vi "Home.vi"() -> ()   [LabVIEW 2019]
uses:
  <vilib>/NI/Current Value Table/Type Defs/Single Tag.ctl
  <vilib>/NI/Current Value Table/Type Defs/Data Types.ctl
  <vilib>/Utility/miscctls.llb/LVDateTimeRec.ctl
  <vilib>/Utility/miscctls.llb/LVPointTypeDef.ctl
  <vilib>/NI/STM/TCP/Read Meta Data (TCP Ref).vi
  <vilib>/NI/STM/TCP/Get Connection Reference (TCP).vi
  <vilib>/NI/AMC/Create Single Message.vi
  <vilib>/NI/AMC/Update Message Routing Info.vi
  <vilib>/NI/AMC/Read Termination Message.vi
  <vilib>/NI/STM/TCP/Read Meta Data (TCP Clst).vi
  <vilib>/NI/AMC/Send Message.vi
  <vilib>/NI/AMC/Globals.vi
  <vilib>/NI/STM/TCP/Write Message (TCP).vi
  <vilib>/NI/STM/NI STM.lvlib
  <vilib>/NI/Current Value Table/Current Value Table.lvlib
  <vilib>/NI/AMC/AMC.lvlib
panel:
  out "Sulfuric Predip":dbl
  out "Current Step  6":i32 caption="Current Step"
  out "Current Step  5":i32 caption="Current Step"
  out "Current Step  4":i32 caption="Current Step"
  out "Current Step  3":i32 caption="Current Step"
  out "Current Step  2":i32 caption="Current Step"
  out "Current Step":i32
  out "Right Output On 6":bool caption="Right Output On"
  out "Left Output On 6":bool caption="Left Output On"
  out "Right Output On 5":bool caption="Right Output On"
  out "Left Output On 5":bool caption="Left Output On"
  out "Right Output On 4":bool caption="Right Output On"
  out "Left Output On 4":bool caption="Left Output On"
  out "Right Output On 3":bool caption="Right Output On"
  out "Left Output On 3":bool caption="Left Output On"
  out "Right Output On 2":bool caption="Right Output On"
  out "Left Output On 2":bool caption="Left Output On"
  out "Right Output On":bool
  out "Left Output On":bool
  out "Process 3 Accum A*hrs":dbl format="%.3f"
  out "Process 2 Accum A*hrs":dbl format="%.3f"
  out "Process 1 Accum A*hrs":dbl format="%.3f"
  in  "Reset All Chemical counters":bool
  out "Sulfuric P3":dbl
  out "Sulfuric P2":dbl
  out "Sulfuric P1":dbl
  out "Leveler P3":dbl
  out "Leveler P2":dbl
  out "Leveler P1":dbl
  out "Suppressor P3":dbl
  out "Suppressor P2":dbl
  out "Suppressor P1":dbl
  out "SPS P3":dbl
  out "SPS P2":dbl
  out "SPS P1":dbl
  out "Copper Oxide P3":dbl format="%.1f"
  out "Copper Oxide P2":dbl
  out "Copper Oxide P1":dbl format="%.1f"
  out "Since":timestamp
  in  "Reset DI Total counter":bool
  in  "LockOut HMI":bool
  out "User":string
  in  "Logout":bool
  in  "Login":bool
  out "Time Secs":dbl(knob) scale=0.0..12.0
  out "Time Mins":dbl(knob) scale=0.0..12.0
  out "Time Hours":dbl(knob) scale=0.0..12.0
  out "Liters DI Usage":dbl format="%#.1f"
  out "Main Electrical Cabinet T":dbl(slide) scale=10.0..55.0
  in  "Machine":bool
  in  "Run":bool
  in  "Basement 4":bool
  in  "Dryer":bool
  in  "Rinse 4":bool
  in  "Rinse 3":bool
  in  "Rinse 2":bool
  in  "Basement 3":bool
  in  "Basement 2":bool
  in  "Basement 1":bool
  in  "Plater 6":bool
  in  "Plater 5":bool
  in  "Plater 4":bool
  in  "Plater 3":bool
  in  "Plater 2":bool
  in  "Plater 1":bool
  in  "Predip":bool
  in  "Rinse 1":bool
  in  "Cleaner":bool
  in  "Etch":bool
  in  "Alarm History":i32(listbox)=-1
  out "# Alarms":u32
  in  "Alarms":i32(listbox)=-1
  in  "stop":bool
  in  "Reset Alarms":bool
  # "Module Selection"
  # "Do Not Operate"
  # "Warning"
  # "Plating Tank Status"
  # "Step"
  # "Left Anode"
  # "Right Anode"
  # "Tank 1"
  # "Tank 2"
  # "C"
  # "Tank 3"
  # "Tank 4"
  # "Tank 5"
  # "Tank 6"
  # "Copper"
  # "SPS"
  # "Suppressor"
  # "Leveler"
  # "Acid"
  # "Water Usage"
  # "Total Amp*Hrs"
  # "g"
  # "g"
  # "g"
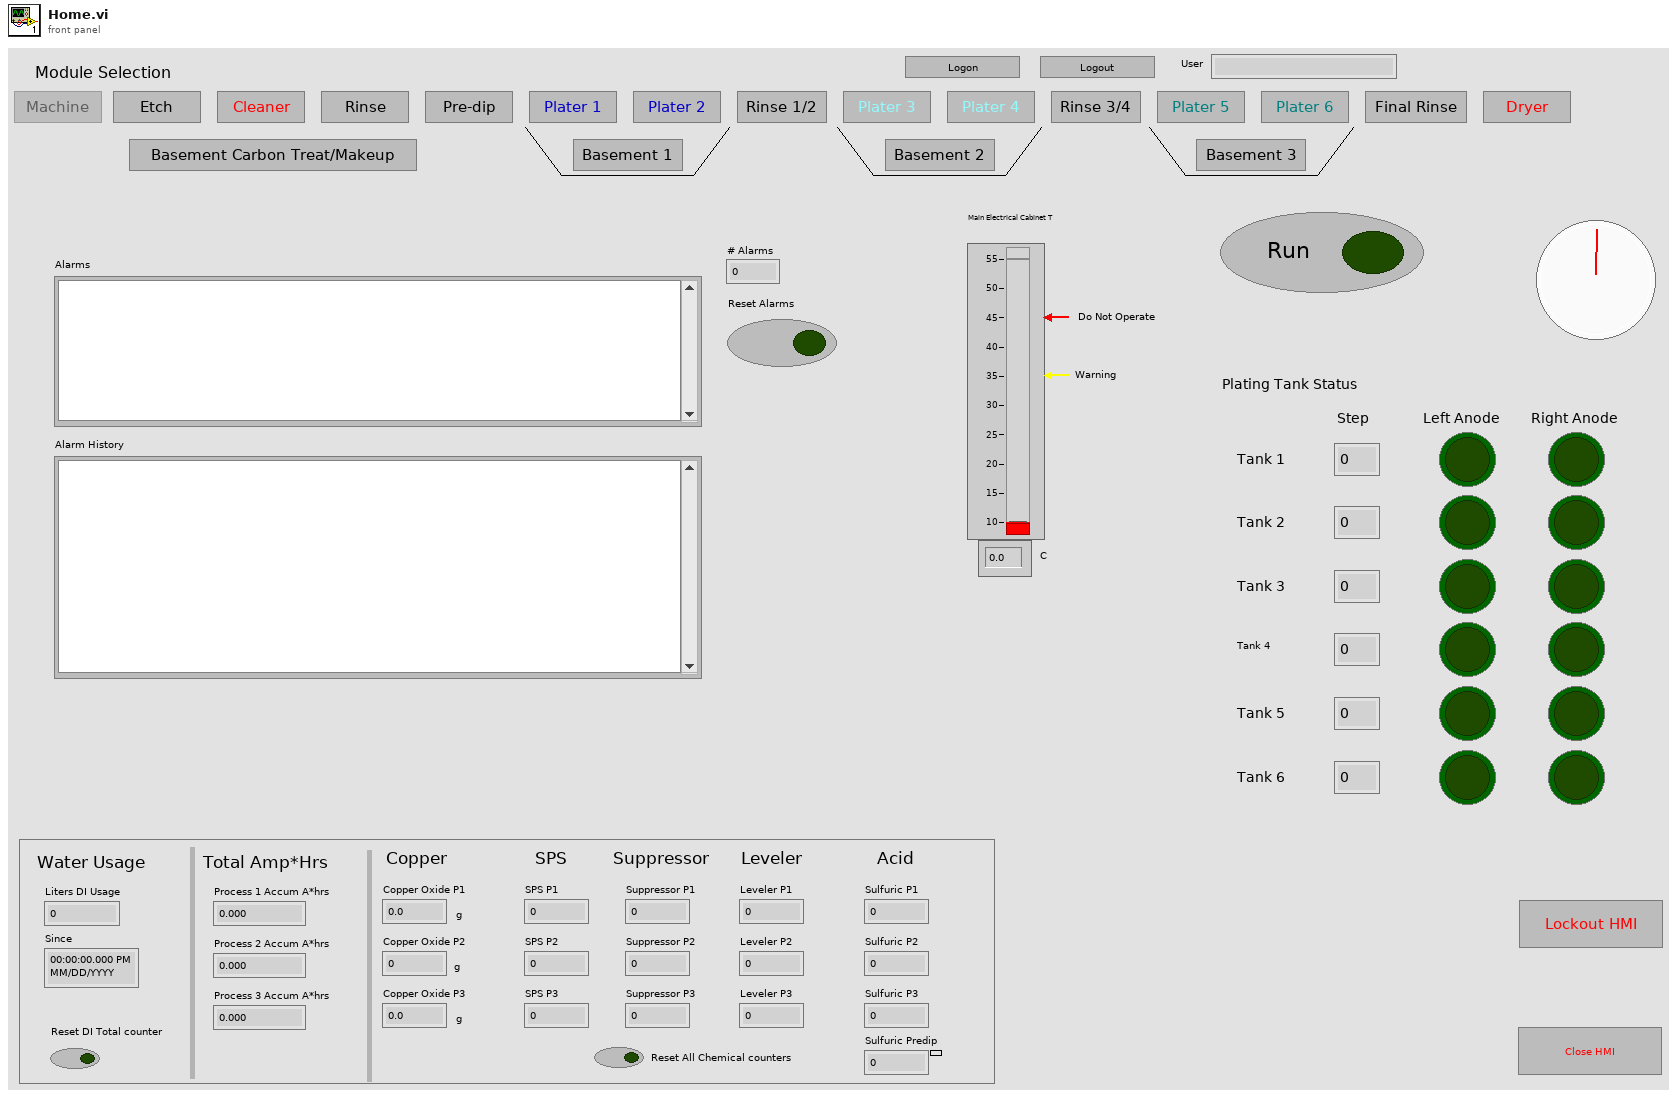
[diagram p1: front panel]
types:
  T1 = typedef "AMC.lvlib/Message Queue.ctl" = refnum<queue>
  T2 = typedef "NI STM.lvlib/TCP Connection Info.ctl" = cluster{"connection ID":refnum<k5>, "meta data":T3[]}
  T3 = typedef "NI STM.lvlib/MetaDataElement.ctl" = string
  T4 = cluster{"Shift":bool, "Ctrl":bool, "Alt":bool, "Cmd":bool, "Opt":bool}
  T5 = typedef "Current Value Table.lvlib/Single Tag.ctl" = cluster{"Data Type":T6, "Name":string, "Value":string, "Description":string}
  T6 = typedef "Current Value Table.lvlib/Data Types.ctl" = enum16{"Double", "Single", "I64", "I32", "I16", "I8", "U64", "U32", "U16", "U8", "String", "Boolean", "Array of U8", "Array of U16", "Array of U32", "Array of U64", "Array of I64", "Array of I32", "Array of I16", "Array of I8", "Array of Double", "Array of Single", "Array of Boolean", "Array of String"}
  T7 = enum8{"Enabled", "Disabled", "Disabled and Grayed Out"}
  T8 = typedef "LVPointTypeDef.ctl" = cluster{"Horizontal":i16, "Vertical":i16}
  T9 = typedef "LVDateTimeRec.ctl" = cluster{"fractional second":dbl, "second":i32, "minute":i32, "hour":i32, "day of month":i32, "month":i32, "year":i32, "day of week":i32, "day of year":i32, "DST":i32}
  T10 = cluster{"second":i32, "minute":i32, "hour":i32, "day of month":i32, "month":i32, "year":i32, "day of week":i32, "day of year":i32, "is DST":i32}
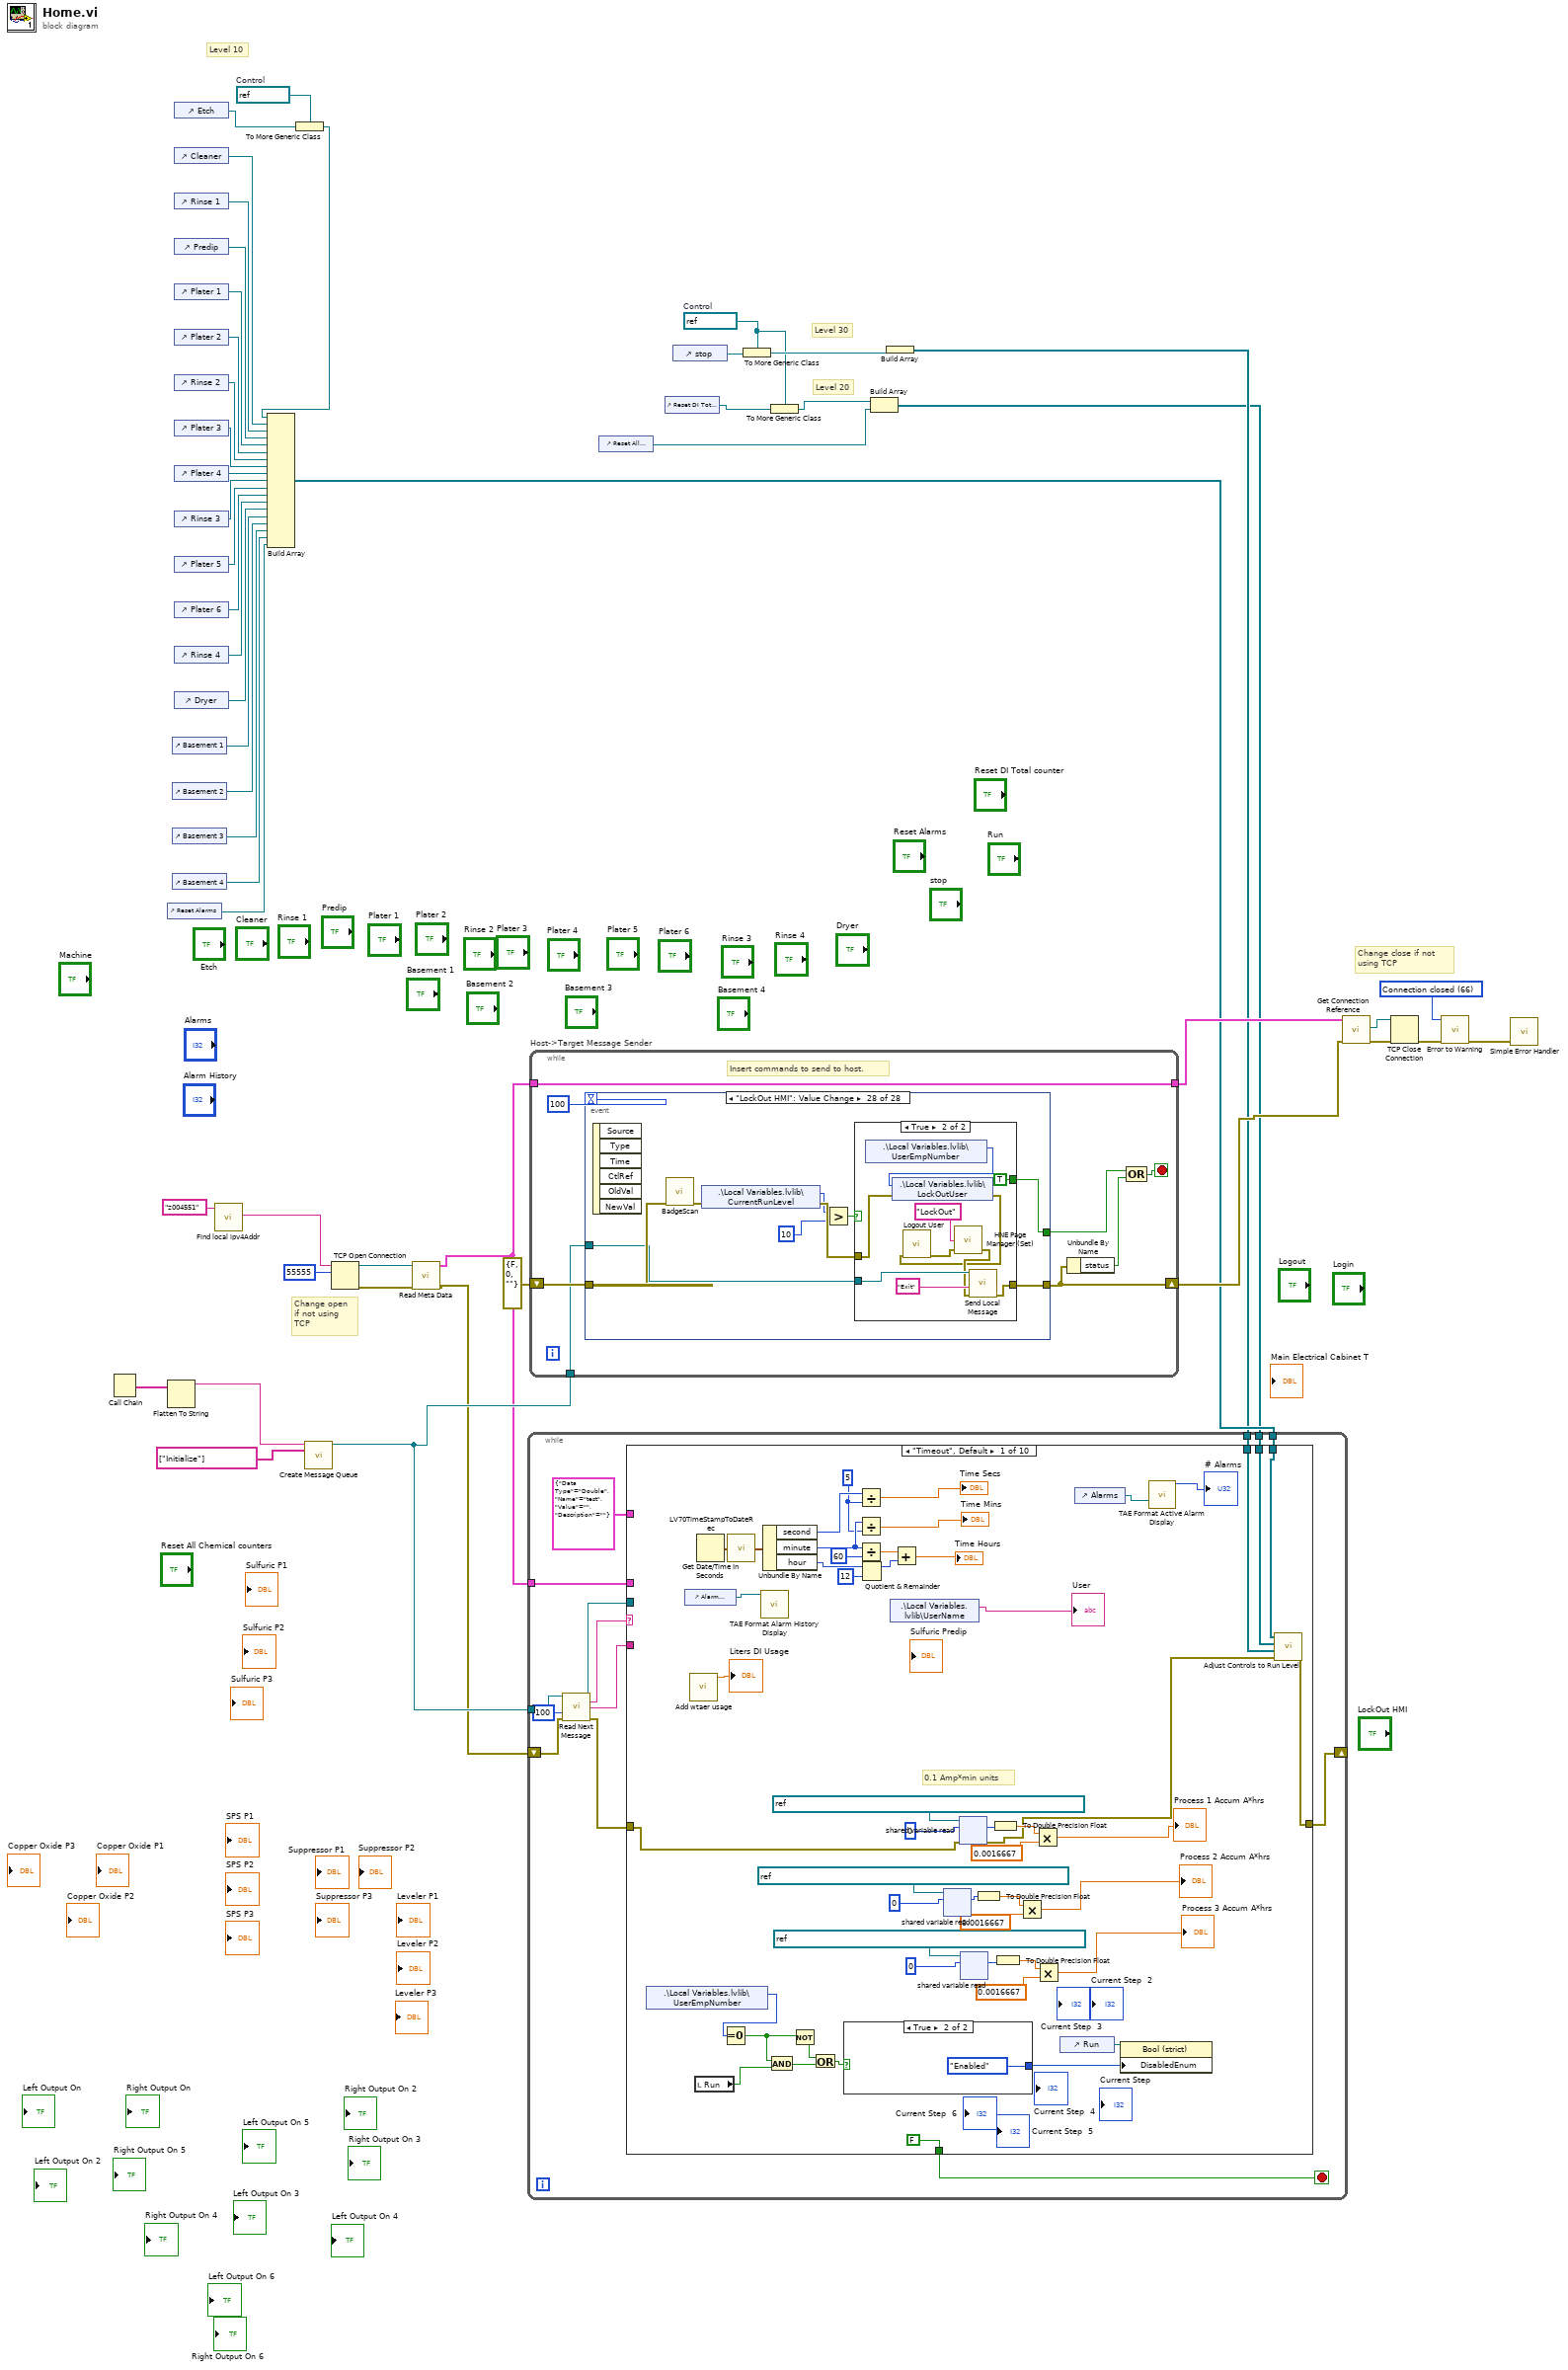
[diagram p0: block diagram]
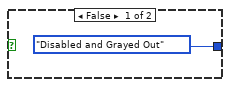
[diagram p2: hidden frame]
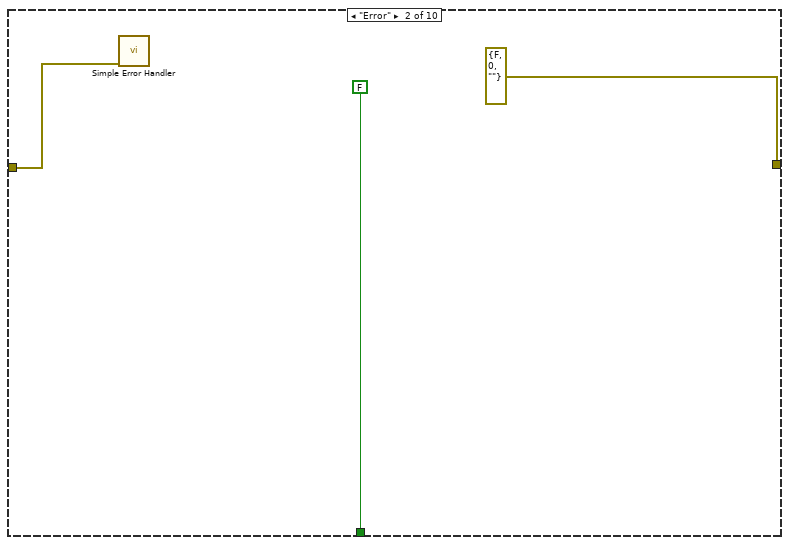
[diagram p3: hidden frame]
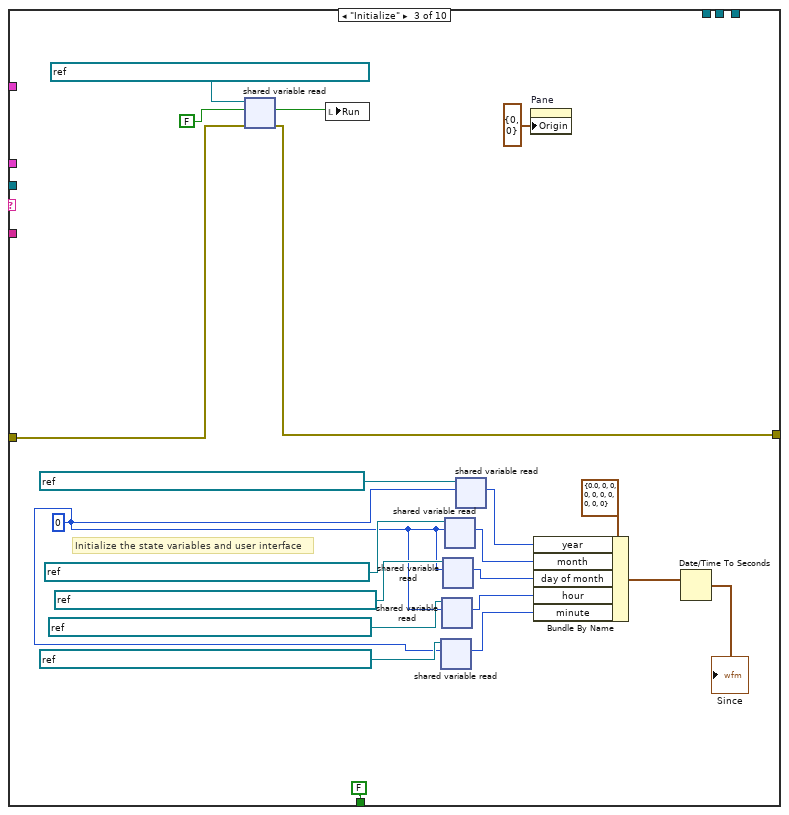
[diagram p4: hidden frame]
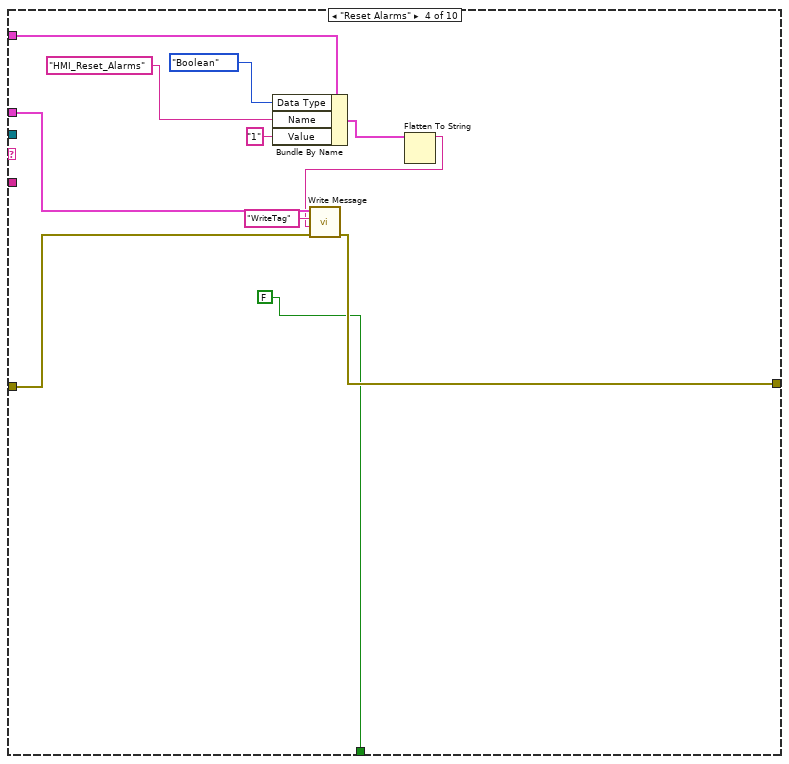
[diagram p5: hidden frame]
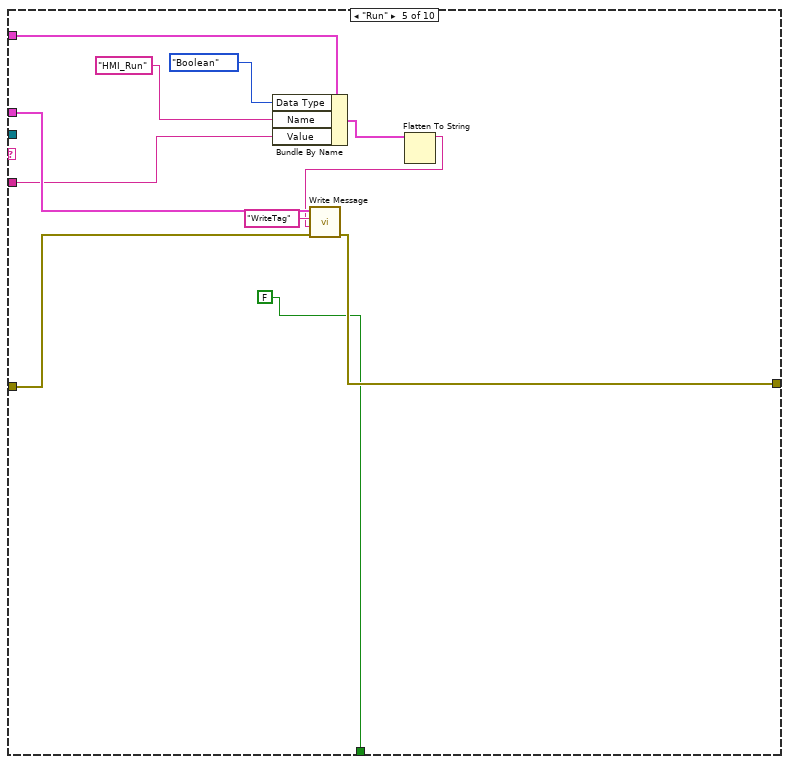
[diagram p6: hidden frame]
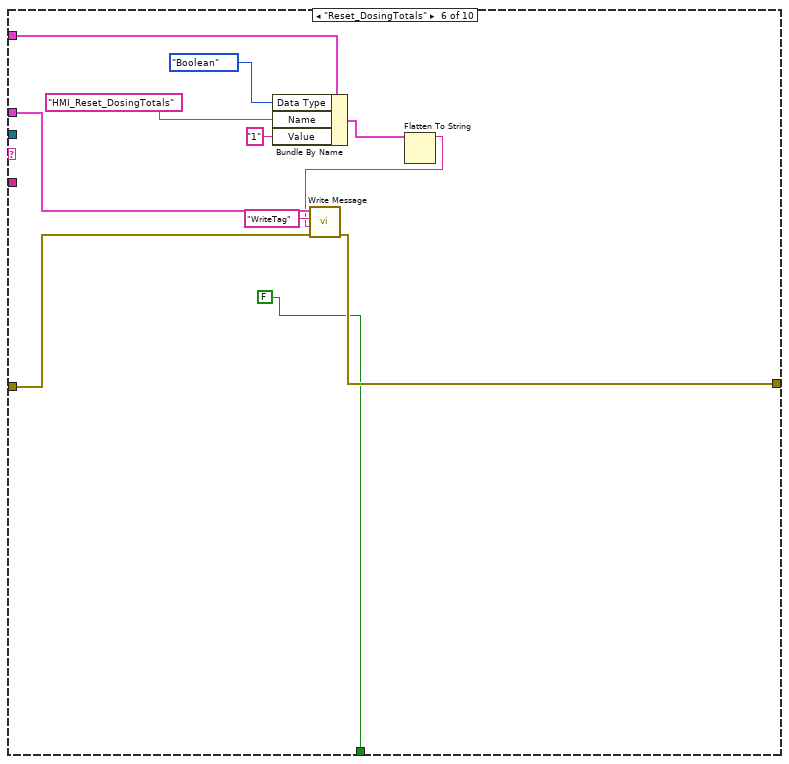
[diagram p7: hidden frame]
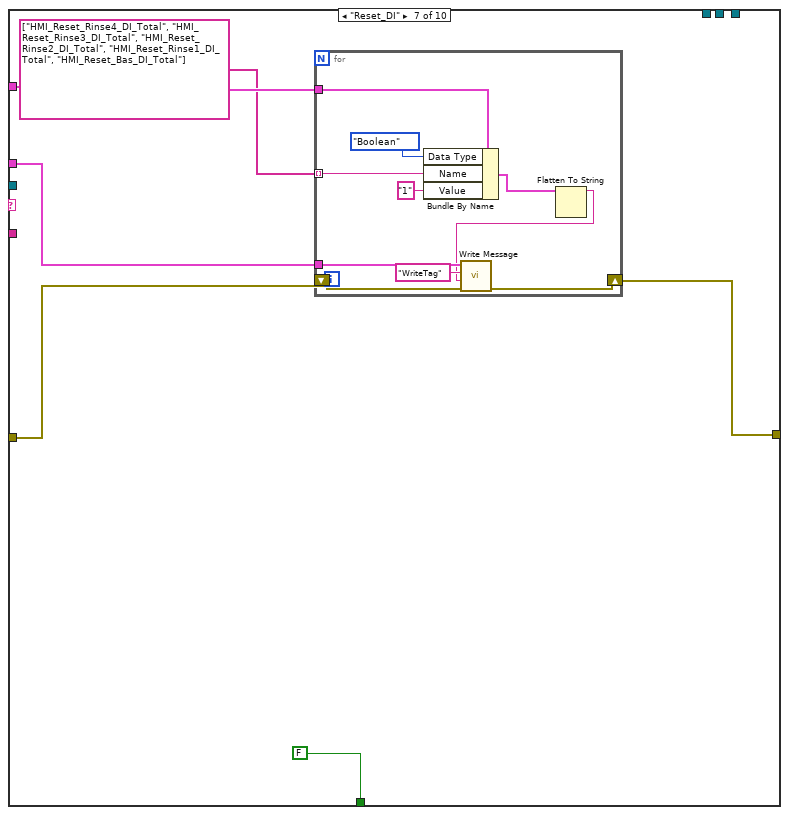
[diagram p8: hidden frame]
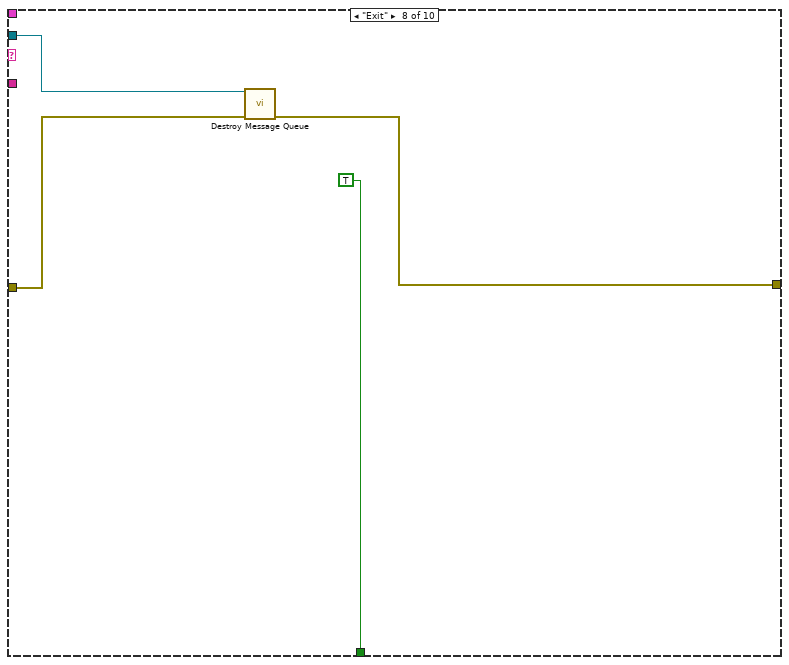
[diagram p9: hidden frame]
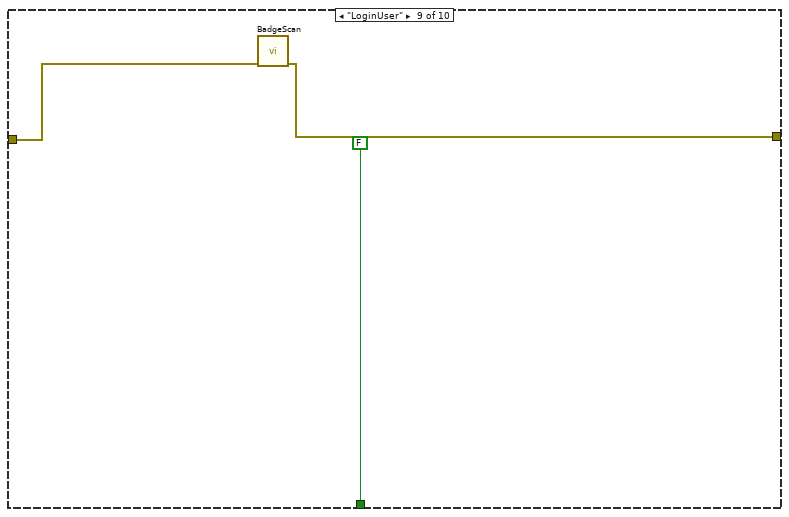
[diagram p10: hidden frame]
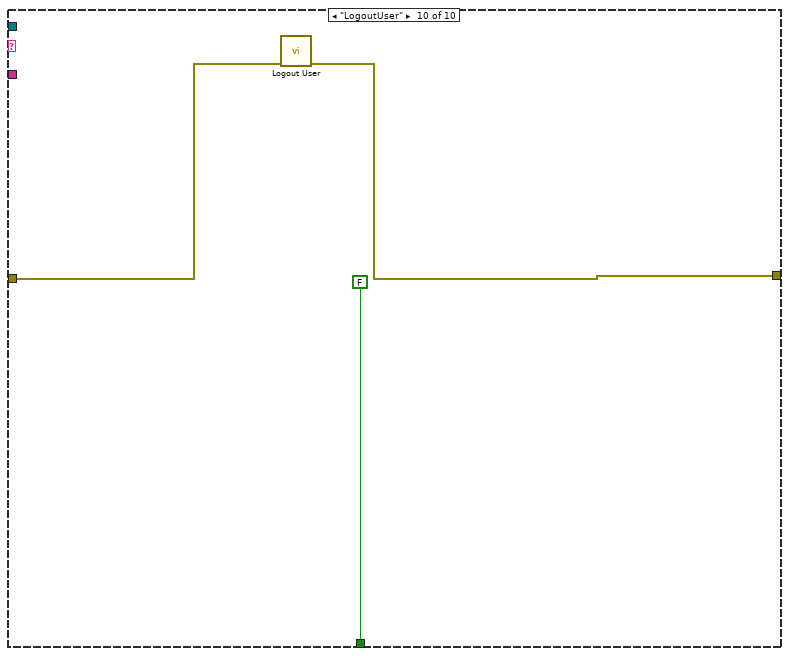
[diagram p11: hidden frame]
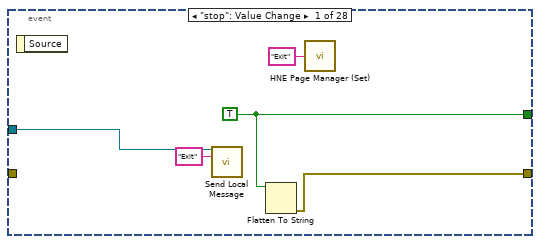
[diagram p12: hidden frame]
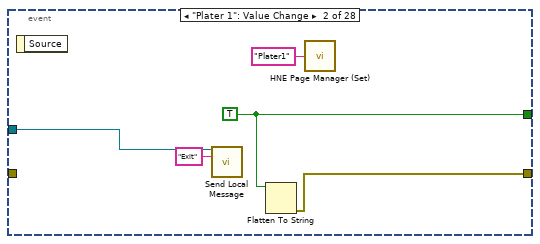
[diagram p13: hidden frame]
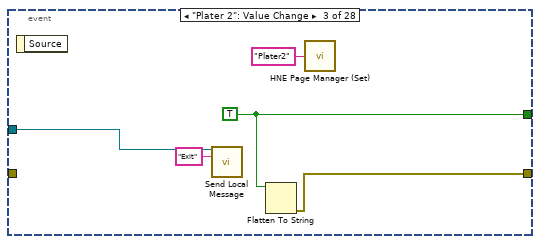
[diagram p14: hidden frame]
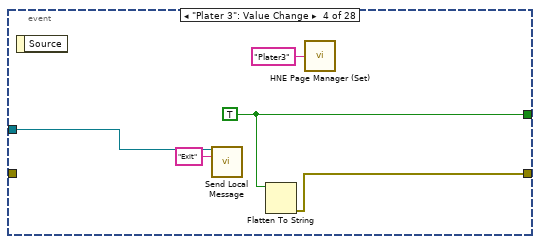
[diagram p15: hidden frame]
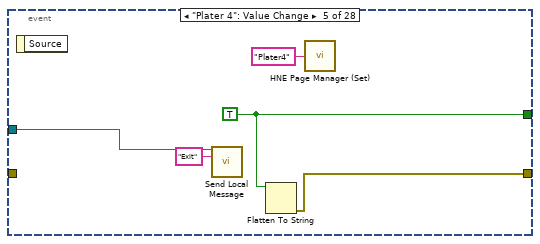
[diagram p16: hidden frame]
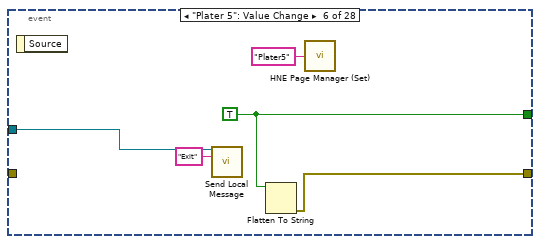
[diagram p17: hidden frame]
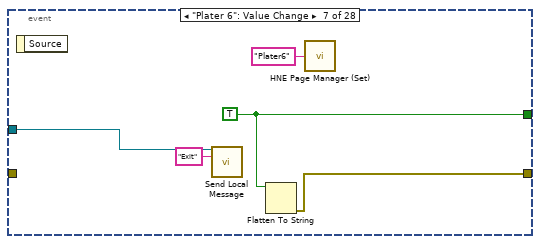
[diagram p18: hidden frame]
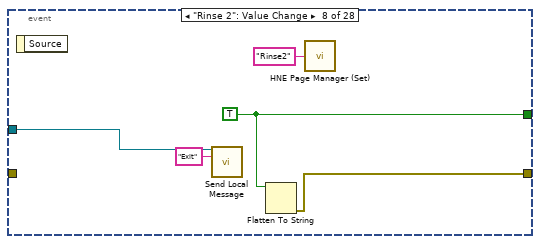
[diagram p19: hidden frame]
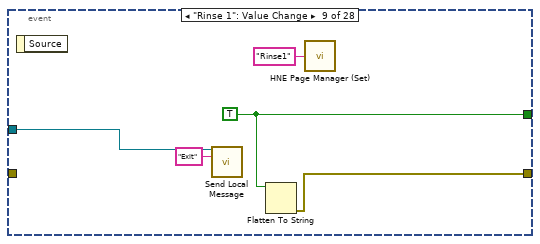
[diagram p20: hidden frame]
diagram:
  w8 = refnum<vi> refnum  # Control
  w4 = refnum<vi> refnum  # Control
  w48 = 66 items=["No Error", "Argument Error", "Memory Full", "Out of Zone", "End of File", "File Already Open", "Generic File IO Error", "File Not Found", "File Permission Error", "Disk Full", "Duplicate Path", "Too Many Files Open", "Not Enabled", "Resource File Not Found", "Cannot Add Resource", "Resource Not Found", "Image Not Found", "Image Memory Error", "Pen Does Not Exist", "Config Bad Type", "Config Token Not Found", "Config Parse Error", "Config Memory Error", "Bad External Code Format", "Bad External Code Offset", "External Code Not Present", "Null Window", "Destroy Window Mixup", "Null Menu", "Print Aborted", "Bad Print Record", "Print Driver Error", "Windows Error During Print", "Memory Error During Print", "Print Dialog Error", "Generic Print Error", "Invalid Device Refnum", "Device Not Found", "Device Parameter Error", "Device Unit Error", "Can't Open Device", "Device Call Aborted", "Generic Error", "Cancelled By User", "Object ID Too Low", "Object ID Too High", "Object Not In Heap", "Unknown Heap", "Bad DefProc ID", "DefProc Not In Table", "Message Out Of Range", "Null Method", "Unknown Message", "Manager Call Not Supported", "Bad address", "Connection In progress", "Connection timed out", "Connection is already in progress", "Network attribute not supported", "Network error", "Address in use", "System out of memory", "Connection aborted", "Connection refused", "Connection is not connected", "Connection is already connected", "Connection closed", "Initialize error (interapplication manager)", "Bad occurrence", "Wait on unbound occurrence handler", "Occurrence queue overflow", "Bad path", "Semaphore not signaled", "Unrecognized type (interapplication manager)"] ("1st Error to Convert")
  # "Level 10"
  # "Level 20"
  # "Level 30"
  # "Change close if not using TCP"
  # "Change open if not using TCP"
  n1 = Call Chain() -> (call chain=w40:string[])
  n2 = control-ref of="Reset Alarms"() -> (w12:refnum<vi>)
  n3 = Flatten To String(anything=w40) -> (data string=w39:string)  [unwired: 3 in, 2 out]
  n4 = control-ref of="Basement 1"() -> (w17:refnum<vi>)
  n5 = control-ref of="Basement 2"() -> (w16:refnum<vi>)
  n6 = control-ref of="Basement 3"() -> (w15:refnum<vi>)
  n7 = control-ref of="Basement 4"() -> (w14:refnum<vi>)
  n8 = control-ref of="Etch"() -> (w7:refnum<vi>)
  n9 = control-ref of="Cleaner"() -> (w30:refnum<vi>)
  n10 = control-ref of="Rinse 1"() -> (w29:refnum<vi>)
  n11 = control-ref of="Predip"() -> (w28:refnum<vi>)
  n12 = control-ref of="Plater 1"() -> (w27:refnum<vi>)
  n13 = control-ref of="Plater 2"() -> (w26:refnum<vi>)
  n14 = control-ref of="Rinse 2"() -> (w25:refnum<vi>)
  n15 = control-ref of="Plater 3"() -> (w24:refnum<vi>)
  n16 = control-ref of="Plater 4"() -> (w23:refnum<vi>)
  n17 = control-ref of="Rinse 3"() -> (w22:refnum<vi>)
  n18 = control-ref of="Plater 5"() -> (w21:refnum<vi>)
  n19 = control-ref of="Plater 6"() -> (w20:refnum<vi>)
  n20 = control-ref of="Rinse 4"() -> (w19:refnum<vi>)
  n21 = control-ref of="Dryer"() -> (w18:refnum<vi>)
  n22 = call "Find local ipv4Addr.vi"("MachineToFind"="z004551") -> ("name"=w34:string)  [unwired: 9 in, 1 out]
  n23 = To More Generic Class(target class=w8, reference=w7) -> (generic class reference=w6:refnum<vi>)
  n24 = Build Array(w6, w30, w29, w28, w27, w26, w25, w24, w23, w22, w21, w20, w19, w18, w17, w16, w15, w14, w12) -> (w13:refnum<vi>[])
  n25 = call <vilib>:"Create Message Queue.vi"("message queue name"=w39, "initial message names"=string[] ["Initialize"] ("initial message values")) -> ("message queue out"=w37:T1)  [unwired: 12 in, 1 out]
  n26 = TCP Open Connection(address=w34, remote port or service name=u16 55555 ("remote port")) -> (connection ID=w44:refnum<k5>, error out=w43:errorcluster)  [unwired: 1 in, 2 out]
  n27 = call-poly <vilib>:"Read Meta Data.vi"("error in"=w43, "connection ID"=w44) -> ("error out"=w36:errorcluster, "connection info out"=w32:T2)  [unwired: 7 in, 1 out]
  n28 = while "Host->Target Message Sender" {
    shift-right: [w54] -> w42
    shift-left: errorcluster {"status"=FALSE, "code"=0, "source"=""} ("error out") -> [w57]
    tunnel: [w50] -> w41
    tunnel: w37 -> [w51]
    tunnel: w32 -> [w50]
    stop <- w55 stop-if-true
    # "Insert commands to send to host."
    n29 = event shown="[27] \"LockOut HMI\": Value Change" {
      selector: _ -> [_ _ _ _ _ _ _ _ _ _ _ _ _ _ _ _ _ _ _ _ _ _ _ _ _ _ _ _]
      dyn-events: _ -> [_ _ _ _ _ _ _ _ _ _ _ _ _ _ _ _ _ _ _ _ _ _ _ _ _ _ _ _]
      timeout: 100 -> [_ _ _ _ _ _ _ _ _ _ _ _ _ _ _ _ _ _ _ _ _ _ _ _ _ _ _ _]
      tunnel: w57 -> [_ _ _ _ _ _ _ _ _ _ _ _ _ _ _ _ _ _ _ w154 w161 w166 w175 w183 w187 w190 w191 w205]
      tunnel: [w62 w67 w72 w77 w82 w87 w92 w97 w102 w107 w112 w117 w122 w127 w132 w137 w142 w147 w152 _ _ _ _ _ _ _ _ w197] -> w53
      tunnel: [w61 w66 w71 w76 w81 w86 w91 w96 w101 w106 w111 w116 w121 w126 w131 w136 w141 w146 w151 w153 w160 w165 w174 w182 w186 w190 w191 w200] -> w54
      tunnel: w51 -> [w59 w64 w69 w74 w79 w84 w89 w94 w99 w104 w109 w114 w119 w124 w129 w134 w139 w144 w149 w156 w163 w167 w176 w185 w189 _ _ w201]
      event "stop": Value Change {
        w62 = TRUE ("stop")
        n30 = event-data() -> ()  [unwired: 2 out]
        n31 = call <vilib>:"Send Local Message.vi"("message queue in"=w59, "message name"="Exit") -> ()  [unwired: 11 in, 3 out]
        n32 = Flatten To String(anything=w62) -> (error out=w61:errorcluster)  [unwired: 2 in, 3 out]
        n33 = call <userlib>:"HNE Page Manager (Set).vi"("Next Page"="Exit") -> ()  [unwired: 4 in, 1 out]
      }
      event "Plater 1": Value Change {
        w67 = TRUE ("stop")
        n34 = event-data() -> ()  [unwired: 2 out]
        n35 = call <vilib>:"Send Local Message.vi"("message queue in"=w64, "message name"="Exit") -> ()  [unwired: 11 in, 3 out]
        n36 = Flatten To String(anything=w67) -> (error out=w66:errorcluster)  [unwired: 2 in, 3 out]
        n37 = call <userlib>:"HNE Page Manager (Set).vi"("Next Page"="Plater1") -> ()  [unwired: 4 in, 1 out]
      }
      event "Plater 2": Value Change {
        w72 = TRUE ("stop")
        n38 = event-data() -> ()  [unwired: 2 out]
        n39 = call <vilib>:"Send Local Message.vi"("message queue in"=w69, "message name"="Exit") -> ()  [unwired: 11 in, 3 out]
        n40 = Flatten To String(anything=w72) -> (error out=w71:errorcluster)  [unwired: 2 in, 3 out]
        n41 = call <userlib>:"HNE Page Manager (Set).vi"("Next Page"="Plater2") -> ()  [unwired: 4 in, 1 out]
      }
      event "Plater 3": Value Change {
        w77 = TRUE ("stop")
        n42 = event-data() -> ()  [unwired: 2 out]
        n43 = call <vilib>:"Send Local Message.vi"("message queue in"=w74, "message name"="Exit") -> ()  [unwired: 11 in, 3 out]
        n44 = Flatten To String(anything=w77) -> (error out=w76:errorcluster)  [unwired: 2 in, 3 out]
        n45 = call <userlib>:"HNE Page Manager (Set).vi"("Next Page"="Plater3") -> ()  [unwired: 4 in, 1 out]
      }
      event "Plater 4": Value Change {
        w82 = TRUE ("stop")
        n46 = event-data() -> ()  [unwired: 2 out]
        n47 = call <vilib>:"Send Local Message.vi"("message queue in"=w79, "message name"="Exit") -> ()  [unwired: 11 in, 3 out]
        n48 = Flatten To String(anything=w82) -> (error out=w81:errorcluster)  [unwired: 2 in, 3 out]
        n49 = call <userlib>:"HNE Page Manager (Set).vi"("Next Page"="Plater4") -> ()  [unwired: 4 in, 1 out]
      }
      event "Plater 5": Value Change {
        w87 = TRUE ("stop")
        n50 = event-data() -> ()  [unwired: 2 out]
        n51 = call <vilib>:"Send Local Message.vi"("message queue in"=w84, "message name"="Exit") -> ()  [unwired: 11 in, 3 out]
        n52 = Flatten To String(anything=w87) -> (error out=w86:errorcluster)  [unwired: 2 in, 3 out]
        n53 = call <userlib>:"HNE Page Manager (Set).vi"("Next Page"="Plater5") -> ()  [unwired: 4 in, 1 out]
      }
      event "Plater 6": Value Change {
        w92 = TRUE ("stop")
        n54 = event-data() -> ()  [unwired: 2 out]
        n55 = call <vilib>:"Send Local Message.vi"("message queue in"=w89, "message name"="Exit") -> ()  [unwired: 11 in, 3 out]
        n56 = Flatten To String(anything=w92) -> (error out=w91:errorcluster)  [unwired: 2 in, 3 out]
        n57 = call <userlib>:"HNE Page Manager (Set).vi"("Next Page"="Plater6") -> ()  [unwired: 4 in, 1 out]
      }
      event "Rinse 2": Value Change {
        w97 = TRUE ("stop")
        n58 = event-data() -> ()  [unwired: 2 out]
        n59 = call <vilib>:"Send Local Message.vi"("message queue in"=w94, "message name"="Exit") -> ()  [unwired: 11 in, 3 out]
        n60 = Flatten To String(anything=w97) -> (error out=w96:errorcluster)  [unwired: 2 in, 3 out]
        n61 = call <userlib>:"HNE Page Manager (Set).vi"("Next Page"="Rinse2") -> ()  [unwired: 4 in, 1 out]
      }
      event "Rinse 1": Value Change {
        w102 = TRUE ("stop")
        n62 = event-data() -> ()  [unwired: 2 out]
        n63 = call <vilib>:"Send Local Message.vi"("message queue in"=w99, "message name"="Exit") -> ()  [unwired: 11 in, 3 out]
        n64 = Flatten To String(anything=w102) -> (error out=w101:errorcluster)  [unwired: 2 in, 3 out]
        n65 = call <userlib>:"HNE Page Manager (Set).vi"("Next Page"="Rinse1") -> ()  [unwired: 4 in, 1 out]
      }
      event "Rinse 3": Value Change {
        w107 = TRUE ("stop")
        n66 = event-data() -> ()  [unwired: 2 out]
        n67 = call <vilib>:"Send Local Message.vi"("message queue in"=w104, "message name"="Exit") -> ()  [unwired: 11 in, 3 out]
        n68 = Flatten To String(anything=w107) -> (error out=w106:errorcluster)  [unwired: 2 in, 3 out]
        n69 = call <userlib>:"HNE Page Manager (Set).vi"("Next Page"="Rinse3") -> ()  [unwired: 4 in, 1 out]
      }
      event "Rinse 4": Value Change {
        w112 = TRUE ("stop")
        n70 = event-data() -> ()  [unwired: 2 out]
        n71 = call <vilib>:"Send Local Message.vi"("message queue in"=w109, "message name"="Exit") -> ()  [unwired: 11 in, 3 out]
        n72 = Flatten To String(anything=w112) -> (error out=w111:errorcluster)  [unwired: 2 in, 3 out]
        n73 = call <userlib>:"HNE Page Manager (Set).vi"("Next Page"="Rinse4") -> ()  [unwired: 4 in, 1 out]
      }
      event "Dryer": Value Change {
        w117 = TRUE ("stop")
        n74 = event-data() -> ()  [unwired: 2 out]
        n75 = call <vilib>:"Send Local Message.vi"("message queue in"=w114, "message name"="Exit") -> ()  [unwired: 11 in, 3 out]
        n76 = Flatten To String(anything=w117) -> (error out=w116:errorcluster)  [unwired: 2 in, 3 out]
        n77 = call <userlib>:"HNE Page Manager (Set).vi"("Next Page"="Dryer") -> ()  [unwired: 4 in, 1 out]
      }
      event "Predip": Value Change {
        w122 = TRUE ("stop")
        n78 = event-data() -> ()  [unwired: 2 out]
        n79 = call <vilib>:"Send Local Message.vi"("message queue in"=w119, "message name"="Exit") -> ()  [unwired: 11 in, 3 out]
        n80 = Flatten To String(anything=w122) -> (error out=w121:errorcluster)  [unwired: 2 in, 3 out]
        n81 = call <userlib>:"HNE Page Manager (Set).vi"("Next Page"="Predip") -> ()  [unwired: 4 in, 1 out]
      }
      event "Cleaner": Value Change {
        w127 = TRUE ("stop")
        n82 = event-data() -> ()  [unwired: 2 out]
        n83 = call <vilib>:"Send Local Message.vi"("message queue in"=w124, "message name"="Exit") -> ()  [unwired: 11 in, 3 out]
        n84 = Flatten To String(anything=w127) -> (error out=w126:errorcluster)  [unwired: 2 in, 3 out]
        n85 = call <userlib>:"HNE Page Manager (Set).vi"("Next Page"="Clean") -> ()  [unwired: 4 in, 1 out]
      }
      event "Etch": Value Change {
        w132 = TRUE ("stop")
        n86 = event-data() -> ()  [unwired: 2 out]
        n87 = call <vilib>:"Send Local Message.vi"("message queue in"=w129, "message name"="Exit") -> ()  [unwired: 11 in, 3 out]
        n88 = Flatten To String(anything=w132) -> (error out=w131:errorcluster)  [unwired: 2 in, 3 out]
        n89 = call <userlib>:"HNE Page Manager (Set).vi"("Next Page"="Etch") -> ()  [unwired: 4 in, 1 out]
      }
      event "Basement 1": Value Change {
        w137 = TRUE ("stop")
        n90 = event-data() -> ()  [unwired: 2 out]
        n91 = call <vilib>:"Send Local Message.vi"("message queue in"=w134, "message name"="Exit") -> ()  [unwired: 11 in, 3 out]
        n92 = Flatten To String(anything=w137) -> (error out=w136:errorcluster)  [unwired: 2 in, 3 out]
        n93 = call <userlib>:"HNE Page Manager (Set).vi"("Next Page"="Basement1") -> ()  [unwired: 4 in, 1 out]
      }
      event "Basement 2": Value Change {
        w142 = TRUE ("stop")
        n94 = event-data() -> ()  [unwired: 2 out]
        n95 = call <vilib>:"Send Local Message.vi"("message queue in"=w139, "message name"="Exit") -> ()  [unwired: 11 in, 3 out]
        n96 = Flatten To String(anything=w142) -> (error out=w141:errorcluster)  [unwired: 2 in, 3 out]
        n97 = call <userlib>:"HNE Page Manager (Set).vi"("Next Page"="Basement2") -> ()  [unwired: 4 in, 1 out]
      }
      event "Basement 3": Value Change {
        w147 = TRUE ("stop")
        n98 = event-data() -> ()  [unwired: 2 out]
        n99 = call <vilib>:"Send Local Message.vi"("message queue in"=w144, "message name"="Exit") -> ()  [unwired: 11 in, 3 out]
        n100 = Flatten To String(anything=w147) -> (error out=w146:errorcluster)  [unwired: 2 in, 3 out]
        n101 = call <userlib>:"HNE Page Manager (Set).vi"("Next Page"="Basement3") -> ()  [unwired: 4 in, 1 out]
      }
      event "Basement 4": Value Change {
        w152 = TRUE ("stop")
        n102 = event-data() -> ()  [unwired: 2 out]
        n103 = call <vilib>:"Send Local Message.vi"("message queue in"=w149, "message name"="Exit") -> ()  [unwired: 11 in, 3 out]
        n104 = Flatten To String(anything=w152) -> (error out=w151:errorcluster)  [unwired: 2 in, 3 out]
        n105 = call <userlib>:"HNE Page Manager (Set).vi"("Next Page"="Basement4") -> ()  [unwired: 4 in, 1 out]
      }
      event "Reset Alarms": Value Change {
        n106 = event-data() -> ()  [unwired: 2 out]
        n107 = call <vilib>:"Send Local Message.vi"("message queue in"=w156, "message name"="Reset Alarms", "error in"=w154) -> ("error out"=w153:errorcluster)  [unwired: 10 in, 2 out]
      }
      event "Run": Value Change {
        n108 = event-data() -> ("NewVal"=w159:bool)  [unwired: 1 out]
        n109 = Boolean To (0,1)(Boolean=w159) -> (0, 1=w158:i16)
        n110 = Number To Decimal String(number=w158) -> (decimal integer string=w157:string)  [unwired: 1 in]
        n111 = call <vilib>:"Send Local Message.vi"("message queue in"=w163, "message name"="Run", "message value"=w157, "error in"=w161) -> ("error out"=w160:errorcluster)  [unwired: 9 in, 2 out]
      }
      event "Reset DI Total counter": Value Change {
        n112 = event-data() -> ("NewVal"=w164:bool)  [unwired: 1 out]
        n113 = case shown="True" w164 {
          tunnel: w167 -> [_ w172]
          tunnel: w166 -> [w168 w170]
          tunnel: [w168 w169] -> w165
          frame False {
          }
          frame True {
            n114 = call <vilib>:"Send Local Message.vi"("message queue in"=w172, "message name"="Reset_DI", "error in"=w170) -> ("error out"=w169:errorcluster)  [unwired: 10 in, 2 out]
          }
        }
      }
      event "Reset All Chemical counters": Value Change {
        n115 = event-data() -> ("NewVal"=w173:bool)  [unwired: 1 out]
        n116 = case shown="True" w173 {
          tunnel: w176 -> [_ w181]
          tunnel: w175 -> [w177 w179]
          tunnel: [w177 w178] -> w174
          frame False {
          }
          frame True {
            n117 = call <vilib>:"Send Local Message.vi"("message queue in"=w181, "message name"="Reset_DosingTotals", "error in"=w179) -> ("error out"=w178:errorcluster)  [unwired: 10 in, 2 out]
          }
        }
      }
      event "Login": Value Change {
        n118 = event-data() -> ()  [unwired: 7 out]
        n119 = call <vilib>:"Send Local Message.vi"("message queue in"=w185, "message name"="LoginUser", "error in"=w183) -> ("error out"=w182:errorcluster)  [unwired: 10 in, 2 out]
      }
      event "Logout": Value Change {
        n120 = event-data() -> ()  [unwired: 7 out]
        n121 = call <vilib>:"Send Local Message.vi"("message queue in"=w189, "message name"="LogoutUser", "error in"=w187) -> ("error out"=w186:errorcluster)  [unwired: 10 in, 2 out]
      }
      event Timeout {
        n122 = event-data() -> ()  [unwired: 2 out]
      }
      event Mouse Down? {
        n123 = event-data() -> ("Button"=w196:u16, "Mods"=w195:cluster{"Double Click":bool, "Menu Key":bool}, "PlatMods"=w194:T4)  [unwired: 6 out]
        n124 = Get Date/Time In Seconds() -> (seconds since 1Jan1904=w192:timestamp)
        n125 = shared-variable ".\\Local Variables.lvlib\\LastLogonTime"(w192) -> ()  [unwired: 1 in, 1 out]
        n126 = event-data("Button"=w196, "Mods"=w195, "PlatMods"=w194, "Discard?"=FALSE) -> ()  [unwired: 1 in, 1 out]
      }
      event "LockOut HMI": Value Change {
        n127 = event-data() -> ()  [unwired: 7 out]
        n128 = call "BadgeScan.vi"("error in"=w205) -> ("error out"=w204:errorcluster)  [unwired: 10 in]
        n129 = shared-variable ".\\Local Variables.lvlib\\CurrentRunLevel"(error in=w204) -> (w199:i32, error out=w202:errorcluster)
        n130 = Greater?(x=w199, y=10 ("x")) -> (0:w203:bool)
        n131 = case shown="True" w203 {
          tunnel: w202 -> [w207 w210]
          tunnel: w201 -> [_ w216]
          tunnel: [w207 w214] -> w200
          tunnel: [FALSE ("stop") TRUE ("stop")] -> w197
          frame False {
          }
          frame True {
            n132 = shared-variable ".\\Local Variables.lvlib\\UserEmpNumber"() -> (w211:i32)  [unwired: 1 in, 1 out]
            n133 = shared-variable ".\\Local Variables.lvlib\\LockOutUser"(w211, error in=w210) -> (error out=w209:errorcluster)
            n134 = call "Logout User.vi"("error in (no error)"=w209) -> ("error out"=w212:errorcluster)  [unwired: 10 in]
            n135 = call <userlib>:"HNE Page Manager (Set).vi"("error in (no error)"=w212, "Next Page"="LockOut") -> ("error out"=w213:errorcluster)  [unwired: 3 in]
            n136 = call <vilib>:"Send Local Message.vi"("message queue in"=w216, "message name"="Exit", "error in"=w213) -> ("error out"=w214:errorcluster)  [unwired: 10 in, 2 out]
          }
        }
      }
    }
    n137 = Unbundle By Name(w54) -> ("status"=w52:bool)
    n138 = Compound Arithmetic op=OR(w53, w52) -> (w55:bool)
  }
  n139 = control-ref of="Reset All Chemical counters"() -> (w1:refnum<vi>)
  n140 = control-ref of="Reset DI Total counter"() -> (w5:refnum<vi>)
  n141 = control-ref of="stop"() -> (w11:refnum<vi>)
  n142 = To More Generic Class(target class=w4, reference=w11) -> (generic class reference=w10:refnum<vi>)
  n143 = To More Generic Class(target class=w4, reference=w5) -> (generic class reference=w3:refnum<vi>)
  n144 = Build Array(w3, w1) -> (w2:refnum<vi>[])
  n145 = Build Array(w10) -> (w9:refnum<vi>[])
  n146 = while {
    tunnel: w37 -> [w231]
    tunnel: w32 -> [w228]
    shift-right: [w226] -> _
    shift-left: w36 -> [w222]
    tunnel: w13 -> [w220]
    tunnel: w9 -> [w219]
    tunnel: w2 -> [w218]
    stop <- w225 stop-if-true
    n147 = call <vilib>:"Read Next Message.vi"("message queue in"=w231, "timeout (1 ms)"=100, "error in"=w222) -> ("message queue out"=w224:T1, "message name"=w229:string, "message value"=w227:string, "error out"=w221:errorcluster)  [unwired: 5 in, 4 out]
    n148 = case shown="\"Timeout\", Default" w229 {
      tunnel: w228 -> [_ _ _ w318 w329 w340 w347 _ _ _]
      tunnel: w227 -> [_ _ _ _ w320 _ _ _ _ _]
      tunnel: w221 -> [w233 w285 w305 w317 w328 w339 w346 w359 w364 w366]
      tunnel: [w234 errorcluster {"status"=FALSE, "code"=0, "source"=""} ("error out") w304 w316 w327 w338 w345 w358 w363 w365] -> w226
      tunnel: [FALSE FALSE FALSE FALSE FALSE FALSE FALSE TRUE FALSE FALSE] -> w225
      tunnel: w224 -> [_ _ _ _ _ _ _ w360 _ _]
      tunnel: T5 {"Data Type"=enum."Double", "Name"="test", "Value"="", "Description"=""} ("Tag") -> [_ _ _ w310 w322 w333 w344 _ _ _]
      tunnel: w220 -> [w255 _ _ _ _ _ _ _ _ _]
      tunnel: w219 -> [w254 _ _ _ _ _ _ _ _ _]
      tunnel: w218 -> [w253 _ _ _ _ _ _ _ _ _]
      frame "Timeout", Default {
        w269 = 5 ("y")
        # "0.1 Amp*min units"
        n149 = shared-variable ".\\Local Variables.lvlib\\UserEmpNumber"() -> (w263:i32)  [unwired: 1 in, 1 out]
        n150 = control-ref of="Alarm History"() -> (w279:refnum<vi>)
        n151 = call "Add wtaer usage.vi"() -> ("Numeric"=→"Liters DI Usage":dbl)  [unwired: 11 in]
        n152 = local read "Run"() -> (w262:bool)
        n153 = Get Date/Time In Seconds() -> (seconds since 1Jan1904=w268:timestamp)
        n154 = Equal To 0?(x=w263) -> (x = 0?=w261:bool)
        n155 = call <vilib>:"LV70TimeStampToDateRec.vi"("time stamp"=w268) -> ("date time rec"=w277:T10)
        n156 = call <userlib>:"TAE Format Alarm History Display.vi"("List Box Ref"=w279) -> ()  [unwired: 13 in, 2 out]
        n157 = Unbundle By Name(w277) -> ("second"=w276:i32, "minute"=w275:i32, "hour"=w272:i32)
        n158 = And(x=w261, y=w262) -> (x .and. y?=w258:bool)
        n159 = Not(x=w261) -> (.not. x?=w259:bool)
        n160 = Or(x=w259, y=w258) -> (x .or. y?=w260:bool)
        n161 = case shown="True" w260 {
          tunnel: [T7."Disabled and Grayed Out" ("Disabled") T7."Enabled" ("Disabled")] -> w256
          frame False {
          }
          frame True {
          }
        }
        n162 = Divide(x=w276, y=w269) -> (x/y=→"Time Secs":dbl)
        n163 = Divide(x=w275, y=w269) -> (x/y=→"Time Mins":dbl)
        n164 = Divide(x=w275, y=60) -> (x/y=w273:dbl)
        n165 = Quotient & Remainder(x=w272, y=12) -> (x-y*floor(x/y)=w270:i32)  [unwired: 1 out]
        n166 = shared-variable ".\\Local Variables.lvlib\\UserName"() -> (→"User":string)  [unwired: 1 in, 1 out]
        n167 = Add(x=w273, y=w270) -> (x+y=→"Time Hours":dbl)
        n168 = shared-variable-read(refnum<k21> "ni.var.psp://z004551/CDL0100 ReadTags/Proc2_TotalAmpMin" ("shared variable refnum in"), 0) -> (w238:i32)  [unwired: 1 in, 3 out]
        n169 = shared-variable-read(refnum<k21> "ni.var.psp://z004551/CDL0100 ReadTags/Proc1_TotalAmpMin" ("shared variable refnum in"), w233, 0) -> (w232:errorcluster, w240:i32)  [unwired: 2 out]
        n170 = shared-variable-read(refnum<k21> "ni.var.psp://z004551/CDL0100 ReadTags/Proc3_TotalAmpMin" ("shared variable refnum in"), 0) -> (w237:i32)  [unwired: 1 in, 3 out]
        n171 = To Double Precision Float(number=w238) -> (double precision float=w235:dbl)
        n172 = To Double Precision Float(number=w240) -> (double precision float=w239:dbl)
        n173 = To Double Precision Float(number=w237) -> (double precision float=w236:dbl)
        n174 = Multiply(x=w235, y=0.0016667) -> (x*y=→"Process 2 Accum A*hrs":dbl)
        n175 = Multiply(x=w239, y=0.0016667) -> (x*y=→"Process 1 Accum A*hrs":dbl)
        n176 = Multiply(x=w236, y=0.0016667) -> (x*y=→"Process 3 Accum A*hrs":dbl)
        n177 = control-ref of="Run"() -> (w257:refnum<vi>)
        n178 = control-ref of="Alarms"() -> (w281:refnum<vi>)
        n179 = property class="Bool (strict)"(reference=w257, "DisabledEnum"=w256) -> ()  [unwired: 1 in, 2 out]
        n180 = call <userlib>:"TAE Format Active Alarm Display.vi"("List Box Ref"=w281) -> ("# Alarms"=→"# Alarms":u32)  [unwired: 14 in]
        n181 = call "Adjust Controls to Run Level.vi"("error in (no error)"=w232, "Level 30 Controls"=w254, "Level 20 Controls"=w253, "Level 10 Controls"=w255) -> ("error out"=w234:errorcluster)  [unwired: 7 in]
      }
      frame "Error" {
        n182 = call <vilib>:"Simple Error Handler.vi"("error in (no error)"=w285) -> ()  [unwired: 4 in, 5 out]
      }
      frame "Initialize" {
        w291 = u32 0
        # "Initialize the state variables and user interface"
        n183 = shared-variable-read(refnum<k21> "ni.var.psp://z004551/CDL0100 ReadWriteTags/HMI_Run" ("shared variable refnum in"), w305, FALSE) -> (w304:errorcluster, w306:bool)  [unwired: 2 out]
        n184 = local write "Run"(w306) -> ()
        n185 = shared-variable-read(refnum<k21> "ni.var.psp://z004551/CDL0100 ReadTags/Rinse1_Reset_Mn" ("shared variable refnum in"), w291) -> (w290:u32)  [unwired: 1 in, 3 out]
        n186 = shared-variable-read(refnum<k21> "ni.var.psp://z004551/CDL0100 ReadTags/Rinse1_Reset_H" ("shared variable refnum in"), w291) -> (w293:u32)  [unwired: 1 in, 3 out]
        n187 = shared-variable-read(refnum<k21> "ni.var.psp://z004551/CDL0100 ReadTags/Rinse1_Reset_D" ("shared variable refnum in"), w291) -> (w295:u32)  [unwired: 1 in, 3 out]
        n188 = shared-variable-read(refnum<k21> "ni.var.psp://z004551/CDL0100 ReadTags/Rinse1_Reset_M" ("shared variable refnum in"), w291) -> (w297:u32)  [unwired: 1 in, 3 out]
        n189 = shared-variable-read(refnum<k21> "ni.var.psp://z004551/CDL0100 ReadTags/Rinse1_Reset_Yr" ("shared variable refnum in"), w291) -> (w299:u32)  [unwired: 1 in, 3 out]
        n190 = property on="Pane" class="Pane"("Origin"=T8 {"Horizontal"=0, "Vertical"=0}) -> ()  [unwired: 2 in, 2 out]
        n191 = Bundle By Name(cluster=T9 {"fractional second"=0.0, "second"=0, "minute"=0, "hour"=0, "day of month"=0, "month"=0, "year"=0, "day of week"=0, "day of year"=0, "DST"=0} ("date time rec"), "year"=w299, "month"=w297, "day of month"=w295, "hour"=w293, "minute"=w290) -> (w301:T9)
        n192 = Date/Time To Seconds(2:w301) -> (0:→"Since":timestamp)  [unwired: 1 in]
      }
      frame "Reset Alarms" {
        n193 = Bundle By Name(cluster=w310, "Data Type"=Data_Types."Boolean", "Name"="HMI_Reset_Alarms", "Value"="1") -> (w311:T5)
        n194 = Flatten To String(anything=w311) -> (data string=w312:string)  [unwired: 3 in, 2 out]
        n195 = call-poly <vilib>:"Write Message.vi"("error in"=w317, "data"=w312, "name"="WriteTag", "connection info in"=w318) -> ("error out"=w316:errorcluster)  [unwired: 6 in, 1 out]
      }
      frame "Run" {
        n196 = Bundle By Name(cluster=w322, "Data Type"=Data_Types."Boolean", "Name"="HMI_Run", "Value"=w320) -> (w323:T5)
        n197 = Flatten To String(anything=w323) -> (data string=w324:string)  [unwired: 3 in, 2 out]
        n198 = call-poly <vilib>:"Write Message.vi"("error in"=w328, "data"=w324, "name"="WriteTag", "connection info in"=w329) -> ("error out"=w327:errorcluster)  [unwired: 6 in, 1 out]
      }
      frame "Reset_DosingTotals" {
        n199 = Bundle By Name(cluster=w333, "Data Type"=Data_Types."Boolean", "Name"="HMI_Reset_DosingTotals", "Value"="1") -> (w334:T5)
        n200 = Flatten To String(anything=w334) -> (data string=w335:string)  [unwired: 3 in, 2 out]
        n201 = call-poly <vilib>:"Write Message.vi"("error in"=w339, "data"=w335, "name"="WriteTag", "connection info in"=w340) -> ("error out"=w338:errorcluster)  [unwired: 6 in, 1 out]
      }
      frame "Reset_DI" {
        n202 = for {
          tunnel: w347 -> [w356]
          tunnel: string[] ["HMI_Reset_Rinse4_DI_Total", "HMI_Reset_Rinse3_DI_Total", "HMI_Reset_Rinse2_DI_Total", "HMI_Reset_Rinse1_DI_Total", "HMI_Reset_Bas_DI_Total"] -> [w352] mode=indexing
          tunnel: w344 -> [w349]
          shift-right: [w354] -> w345
          shift-left: w346 -> [w355]
          n203 = Bundle By Name(cluster=w349, "Data Type"=Data_Types."Boolean", "Name"=w352, "Value"="1") -> (w350:T5)
          n204 = Flatten To String(anything=w350) -> (data string=w351:string)  [unwired: 3 in, 2 out]
          n205 = call-poly <vilib>:"Write Message.vi"("error in"=w355, "data"=w351, "name"="WriteTag", "connection info in"=w356) -> ("error out"=w354:errorcluster)  [unwired: 6 in, 1 out]
        }
      }
      frame "Exit" {
        n206 = call <vilib>:"Destroy Message Queue.vi"("message queue in"=w360, "error in"=w359) -> ("error out"=w358:errorcluster)  [unwired: 11 in, 2 out]
      }
      frame "LoginUser" {
        n207 = call "BadgeScan.vi"("error in"=w364) -> ("error out"=w363:errorcluster)  [unwired: 10 in]
      }
      frame "LogoutUser" {
        n208 = call "Logout User.vi"("error in (no error)"=w366) -> ("error out"=w365:errorcluster)  [unwired: 10 in]
      }
    }
  }
  n209 = call-poly <vilib>:"Get Connection Reference.vi"("error in"=w42, "connection info in"=w41) -> ("error out"=w46:errorcluster, "connection ID out"=w45:refnum<k5>)  [unwired: 8 out]
  n210 = TCP Close Connection(connection ID=w45, error in (no error)=w46) -> (error out=w49:errorcluster)  [unwired: 2 out]
  n211 = call <vilib>:"Error to Warning.vi"("1st Error to Convert"=w48, "error in"=w49) -> ("warning out"=w35:errorcluster)  [unwired: 3 in, 10 out]
  n212 = call <vilib>:"Simple Error Handler.vi"("error in (no error)"=w35) -> ()  [unwired: 4 in, 5 out]
